vi "Fetch Waveform.vi"(8 "error in (no error)":errorcluster, 9 "Maximum Time (10000 ms)":u32=10000, 10 "Channel (1: Channel 1)":u16(ring)=1 items=["Channel 1"=1, "Channel 2"=2, "Channel 3"=3, "Channel 4"=4], 11 "VISA resource name":refnum<visa-resource-name>) -> (0 "error out":errorcluster, 2 "Waveform Data":waveform(dbl)(graph), 3 "VISA resource name out":refnum<visa-resource-name>)   [LabVIEW 2011, in "Agilent DSO1000 Series.lvlib"]
doc: "Returns the waveform the oscilloscope acquired for the specified channel. The waveform is from an acquisition that you initiate prior to calling this VI.\n\nYou use the Initiate VI to start an acquisition on the channels that you enable with the Configure Channel VI. The oscilloscope acquires waveforms for the enabled channels concurrently. You must call this VI separately for each enabled channel to obtain the waveforms.\n\nYou can call the Read Waveform VI instead of using low-level VIs.\n\n<B>Note:</B> Use this VI only with other low-level VIs. The high-level VIs automatically incorporate this functionality. This VI does not check the instrument status."
uses:
  <instrlib>/Agilent DSO1000 Series/Agilent DSO1000 Series.lvlib
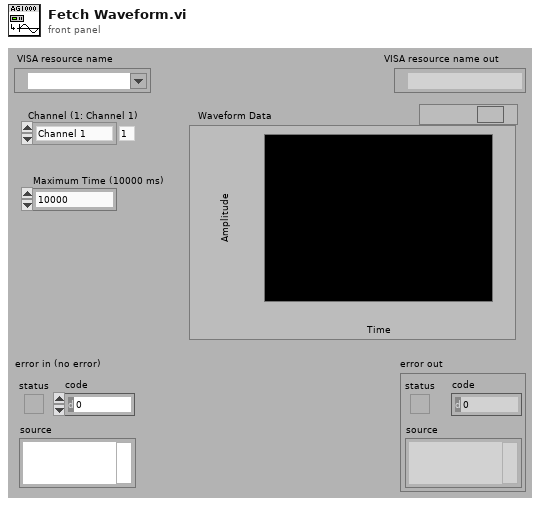
[diagram p1: front panel]
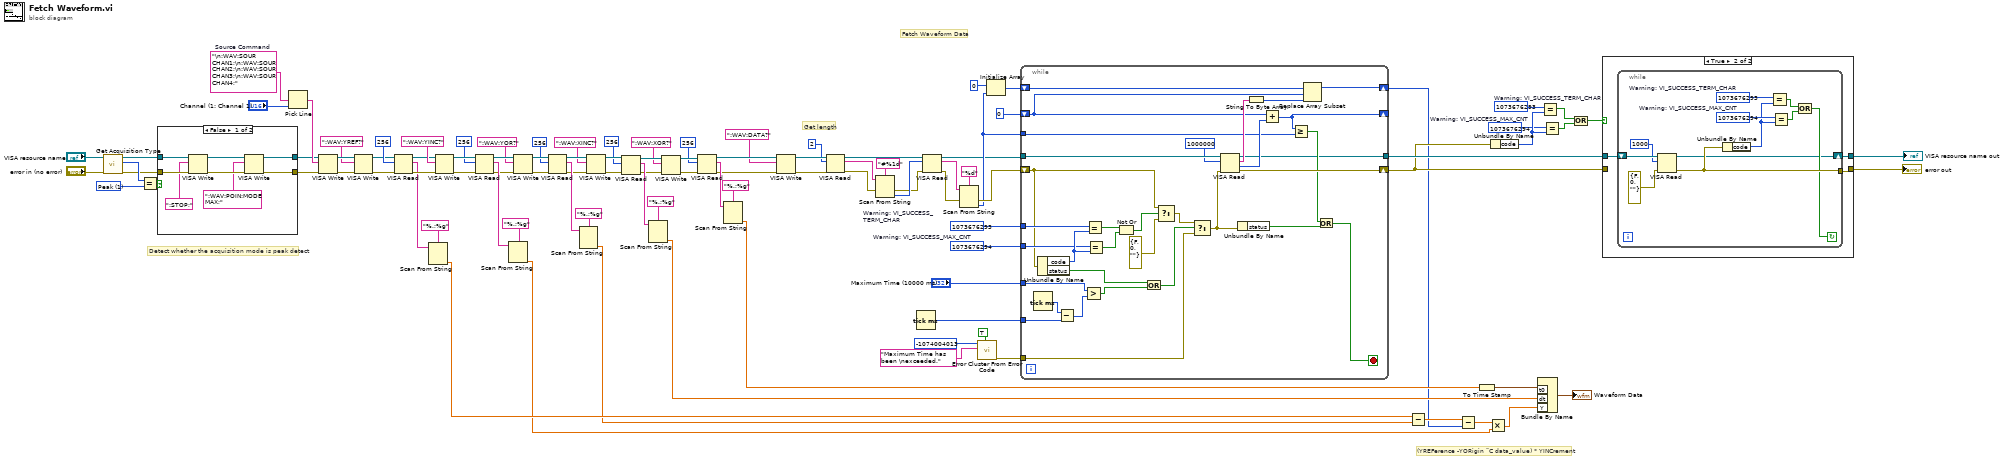
[diagram p0: block diagram]
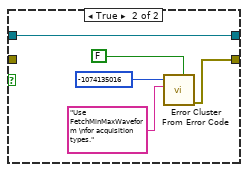
[diagram p2: hidden frame]
diagram:
  w23 = 1 items=["Normal", "Peak", "Average"] ("y")
  w29 = 1073676294  # Warning: VI_SUCCESS_MAX_CNT
  w40 = 1073676293  # Warning: VI_SUCCESS_TERM_CHAR
  w45 = 1073676294  # Warning: VI_SUCCESS_MAX_CNT
  w46 = 1073676293  # Warning: VI_SUCCESS_TERM_CHAR
  w98 = "\n:WAV:SOUR CHAN1;\n:WAV:SOUR CHAN2;\n:WAV:SOUR CHAN3;\n:WAV:SOUR CHAN4;"  # Source Command
  # "(YREFerence -YORigin ¨C data_value) * YINCrement"
  # "Detect whether the acquisition mode is peak detect"
  # "Get length"
  # "Fetch Waveform Data"
  n1 = call <instrlib>:"Get Acquisition Type.vi"("error in (no error)"="error in (no error)", "VISA resource name"="VISA resource name") -> ("error out"=w19:errorcluster, "Acquisition Type"=w24:i32, "VISA resource name out"=w21:refnum<visa-resource-name>)  [unwired: 7 in]
  n2 = Equal?(x=w24, y=w23) -> (x = y?=w22:bool)
  n3 = case shown="False" w22 {
    tunnel: w21 -> [w110 w115]
    tunnel: [w106 w115] -> w20
    tunnel: w19 -> [w109 _]
    tunnel: [w105 w111] -> w18
    frame False {
      n4 = VISA Write(VISA resource name=w110, write buffer=":STOP;", error in (no error)=w109) -> (VISA resource name out=w107:refnum<visa-resource-name>, error out=w104:errorcluster)  [unwired: 1 out]
      n5 = VISA Write(VISA resource name=w107, write buffer=":WAV:POIN:MODE MAX;", error in (no error)=w104) -> (VISA resource name out=w106:refnum<visa-resource-name>, error out=w105:errorcluster)  [unwired: 1 out]
    }
    frame True {
      n6 = call <vilib>:"Error Cluster From Error Code.vi"("is warning? (False)"=FALSE, "error message (\"\")"="Use FetchMinMaxWaveform \nfor acquisition types.", "error code (0)"=-1074135016) -> ("error out"=w111:errorcluster)  [unwired: 6 in]
    }
  }
  n7 = Pick Line(multi-line string=w98, line index="Channel (1: Channel 1)") -> (output string=w101:string)  [unwired: 1 in]
  n8 = VISA Write(VISA resource name=w20, write buffer=w101, error in (no error)=w18) -> (VISA resource name out=w14:refnum<visa-resource-name>, error out=w13:errorcluster)  [unwired: 1 out]
  n9 = VISA Write(VISA resource name=w14, write buffer=":WAV:YREF?", error in (no error)=w13) -> (VISA resource name out=w15:refnum<visa-resource-name>, error out=w16:errorcluster)  [unwired: 1 out]
  n10 = VISA Read(VISA resource name=w15, byte count=u32 256, error in (no error)=w16) -> (VISA resource name out=w11:refnum<visa-resource-name>, read buffer=w8:string, error out=w10:errorcluster)  [unwired: 1 out]
  n11 = Scan From String(format string="%.;%g", input string=w8) -> (output 1=w7:dbl)  [unwired: 3 in, 3 out]
  n12 = VISA Write(VISA resource name=w11, write buffer=":WAV:YINC?", error in (no error)=w10) -> (VISA resource name out=w70:refnum<visa-resource-name>, error out=w69:errorcluster)  [unwired: 1 out]
  n13 = VISA Read(VISA resource name=w70, byte count=u32 256, error in (no error)=w69) -> (VISA resource name out=w95:refnum<visa-resource-name>, read buffer=w97:string, error out=w94:errorcluster)  [unwired: 1 out]
  n14 = Scan From String(format string="%.;%g", input string=w97) -> (output 1=w2:dbl)  [unwired: 3 in, 3 out]
  n15 = VISA Write(VISA resource name=w95, write buffer=":WAV:YOR?", error in (no error)=w94) -> (VISA resource name out=w92:refnum<visa-resource-name>, error out=w91:errorcluster)  [unwired: 1 out]
  n16 = VISA Read(VISA resource name=w92, byte count=u32 256, error in (no error)=w91) -> (VISA resource name out=w87:refnum<visa-resource-name>, read buffer=w89:string, error out=w86:errorcluster)  [unwired: 1 out]
  n17 = Scan From String(format string="%.;%g", input string=w89) -> (output 1=w3:dbl)  [unwired: 3 in, 3 out]
  n18 = VISA Write(VISA resource name=w87, write buffer=":WAV:XINC?", error in (no error)=w86) -> (VISA resource name out=w84:refnum<visa-resource-name>, error out=w83:errorcluster)  [unwired: 1 out]
  n19 = VISA Read(VISA resource name=w84, byte count=u32 256, error in (no error)=w83) -> (VISA resource name out=w79:refnum<visa-resource-name>, read buffer=w81:string, error out=w78:errorcluster)  [unwired: 1 out]
  n20 = Scan From String(format string="%.;%g", input string=w81) -> (output 1=w66:dbl)  [unwired: 3 in, 3 out]
  n21 = VISA Write(VISA resource name=w79, write buffer=":WAV:XOR?", error in (no error)=w78) -> (VISA resource name out=w76:refnum<visa-resource-name>, error out=w75:errorcluster)  [unwired: 1 out]
  n22 = VISA Read(VISA resource name=w76, byte count=u32 256, error in (no error)=w75) -> (VISA resource name out=w31:refnum<visa-resource-name>, read buffer=w73:string, error out=w30:errorcluster)  [unwired: 1 out]
  n23 = Scan From String(format string="%.;%g", input string=w73) -> (output 1=w67:dbl)  [unwired: 3 in, 3 out]
  n24 = VISA Write(VISA resource name=w31, write buffer=":WAV:DATA?" ("multi-line string"), error in (no error)=w30) -> (VISA resource name out=w65:refnum<visa-resource-name>, error out=w64:errorcluster)  [unwired: 1 out]
  n25 = VISA Read(VISA resource name=w65, byte count=u32 2, error in (no error)=w64) -> (VISA resource name out=w60:refnum<visa-resource-name>, read buffer=w61:string, error out=w62:errorcluster)  [unwired: 1 out]
  n26 = Scan From String(format string="#%1d", input string=w61, error in=w62) -> (error out=w57:errorcluster, output 1=w58:i32)  [unwired: 2 in, 2 out]
  n27 = Tick Count (ms)() -> (millisecond timer value=w47:u32)
  n28 = VISA Read(VISA resource name=w60, byte count=w58, error in (no error)=w57) -> (VISA resource name out=w48:refnum<visa-resource-name>, read buffer=w55:string, error out=w56:errorcluster)  [unwired: 1 out]
  n29 = Scan From String(format string="%d", input string=w55, error in=w56) -> (error out=w53:errorcluster, output 1=w49:i32)  [unwired: 2 in, 2 out]
  n30 = call <vilib>:"Error Cluster From Error Code.vi"("show call chain? (False)"=TRUE, "error message (\"\")"="Maximum Time has been \nexceeded." ("error message (\"\")"), "error code (0)"=-1074004013) -> ("error out"=w41:errorcluster)  [unwired: 6 in]
  n31 = Initialize Array(u8 0 ("element"), w49) -> (w51:u8[])
  n32 = while {
    shift-right: [w118] -> w1
    shift-left: w51 -> [w119]
    shift-right: [w126] -> _
    shift-left: 0 ("element") -> [w120]
    tunnel: w49 -> [w125]
    tunnel: w48 -> [w145]
    shift-right: [w129] -> w34
    shift-left: w53 -> [w139]
    tunnel: w47 -> [w148]
    tunnel: w46 -> [w143]
    tunnel: w45 -> [w142]
    tunnel: w41 -> [w132]
    tunnel: [w117] -> w35
    tunnel: "Maximum Time (10000 ms)" -> [w116]
    stop <- w122 stop-if-true
    n33 = Tick Count (ms)() -> (millisecond timer value=w147:u32)
    n34 = Unbundle By Name(w139) -> ("code"=w144:i32, "status"=w135:bool)
    n35 = Subtract(x=w147, y=w148) -> (x-y=w146:u32)
    n36 = Greater?(x=w116, y=w146) -> (0:w136:bool)
    n37 = Equal?(x=w143, y=w144) -> (x = y?=w141:bool)
    n38 = Equal?(x=w142, y=w144) -> (x = y?=w140:bool)
    n39 = Not Or(1:w140, 2:w141) -> (0:w138:bool)
    n40 = Or(x=w135, y=w136) -> (x .or. y?=w134:bool)
    n41 = Select(t=w139, s=w138, f=errorcluster {"status"=FALSE, "code"=0, "source"=""} ("error in (no error) 2")) -> (s? t:f=w133:errorcluster)
    n42 = Select(t=w133, s=w134, f=w132) -> (s? t:f=w131:errorcluster)
    n43 = VISA Read(VISA resource name=w145, byte count=u32 1000000, error in (no error)=w131) -> (VISA resource name out=w117:refnum<visa-resource-name>, read buffer=w128:string, return count=w127:u32, error out=w129:errorcluster)
    n44 = Unbundle By Name(w131) -> ("status"=w123:bool)
    n45 = String To Byte Array(string=w128) -> (unsigned byte array=w121:u8[])
    n46 = Add(x=w120, y=w127) -> (x+y=w126:u32)
    n47 = Greater Or Equal?(x=w126, y=w125) -> (x >= y?=w124:bool)
    n48 = Replace Array Subset(array=w119, new element=w121, index=w120) -> (w118:u8[])
    n49 = Or(x=w124, y=w123) -> (x .or. y?=w122:bool)
  }
  n50 = Subtract(x=w7, y=w3) -> (x-y=w6:dbl)
  n51 = Subtract(x=w6, y=w1) -> (x-y=w5:dbl[])
  n52 = To Time Stamp(1:w67) -> (0:w100:timestamp)
  n53 = Multiply(x=w5, y=w2) -> (x*y=w4:dbl[])
  n54 = Unbundle By Name(w34) -> ("code"=w39:i32)
  n55 = Bundle By Name("t0"=w100, "dt"=w66, "Y"=w4) -> (→"Waveform Data":waveform(dbl))  [unwired: 1 in]
  n56 = Equal?(x=w40, y=w39) -> (x = y?=w38:bool)
  n57 = Equal?(x=w29, y=w39) -> (x = y?=w37:bool)
  n58 = Or(x=w38, y=w37) -> (x .or. y?=w36:bool)
  n59 = case shown="True" w36 {
    tunnel: w35 -> [w150 w153]
    tunnel: w34 -> [w149 _]
    tunnel: [w150 w151] -> w33
    tunnel: [w149 w152] -> w32
    frame False {
    }
    frame True {
      n60 = while {
        shift-right: [w154] -> w151
        shift-left: w153 -> [w164]
        tunnel: [w157] -> w152
        stop <- w155 continue-if-true
        w160 = 1073676294  # Warning: VI_SUCCESS_MAX_CNT
        w161 = 1073676293  # Warning: VI_SUCCESS_TERM_CHAR
        n61 = VISA Read(VISA resource name=w164, byte count=u32 1000, error in (no error)=errorcluster {"status"=FALSE, "code"=0, "source"=""} ("error in (no error) 2")) -> (VISA resource name out=w154:refnum<visa-resource-name>, error out=w157:errorcluster)  [unwired: 2 out]
        n62 = Unbundle By Name(w157) -> ("code"=w156:i32)
        n63 = Equal?(x=w161, y=w156) -> (x = y?=w159:bool)
        n64 = Equal?(x=w160, y=w156) -> (x = y?=w158:bool)
        n65 = Or(x=w159, y=w158) -> (x .or. y?=w155:bool)
      }
    }
  }
  "error out" <- w32
  "VISA resource name out" <- w33
